vi "Stop.vi"(8 "error in (no error)":errorcluster, 11 "NIDIO in":refnum<class "NIDIO.lvclass">) -> (0 "error out":errorcluster, 3 "NIDIO out":refnum<class "NIDIO.lvclass">)   [LabVIEW 2015, in "NIDIO.lvclass"]
uses:
  NIDIO.lvclass
  NIDIO.lvclass/NIDIO.ctl
  DIO.lvclass
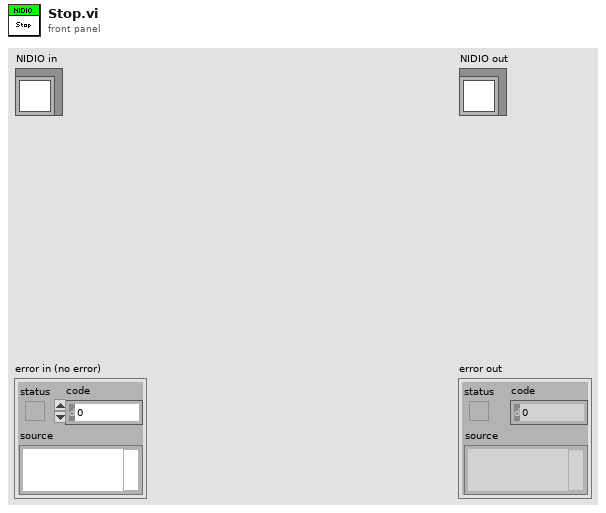
[diagram p1: front panel]
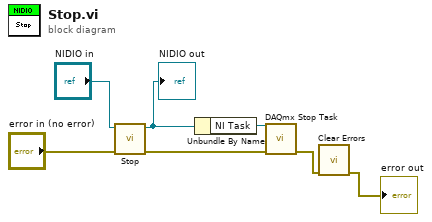
[diagram p0: block diagram]
diagram:
  n1 = call-parent "Stop.vi"("error in (no error)"="error in (no error)", "DIO in"="NIDIO in") -> ("error out"=w5:errorcluster, "DIO out"=w4:refnum<class "NIDIO.lvclass">)  [unwired: 8 in]
  "NIDIO out" <- w4
  n2 = Unbundle By Name(w4) -> ("NI Task"=w3:refnum<k21>)
  n3 = call <vilib>:"DAQmx Stop Task.vi"("task/channels in"=w3, "error in"=w5) -> ("error out"=w2:errorcluster)  [unwired: 12 in, 1 out]
  n4 = call <vilib>:"Clear Errors.vi"("error in (no error)"=w2) -> ("error out"=→"error out":errorcluster)  [unwired: 5 in, 1 out]
